vi "檔案管理.vi"() -> ()   [LabVIEW 2015]
uses:
  Control_cluster_IOConstant.ctl
  C:/Users/jeff.lin.MINAIK/Desktop/Scripting/Control_MessageCluster.ctl
  <userlib>/FGV/control/Control_Data.ctl
panel:
  out "Array 2":string[](array[string])
  in  "Listbox":i32(listbox)
  out "error out":errorcluster
  in  "ProjectName":string
  in  "Project":string(combo)
  in  "file (use dialog)":path=path "D:/dataFGV"
  in  "重新載入":bool
  out "Array":cluster{"Name":string, "Cluster In 2":T1}[](array[cluster])
  in  "Cluster In":T1
  out "Cluster Out":cluster{"Name":string, "Cluster In 2":T1}
  in  "儲存檔案":bool
  in  "匯入檔案":bool
  in  "開啟檔案":bool
  in  "檔案初始化":bool
  in  "更新資料":bool
  in  "刪除資料":bool
  in  "插入資料":bool
  in  "增加資料":bool
  in  "儲存資料":bool
  in  "讀取資料":bool
  in  "資料初始化":bool
  in  "離開":bool
  in  "等待":bool
  in  "系統初始化":bool
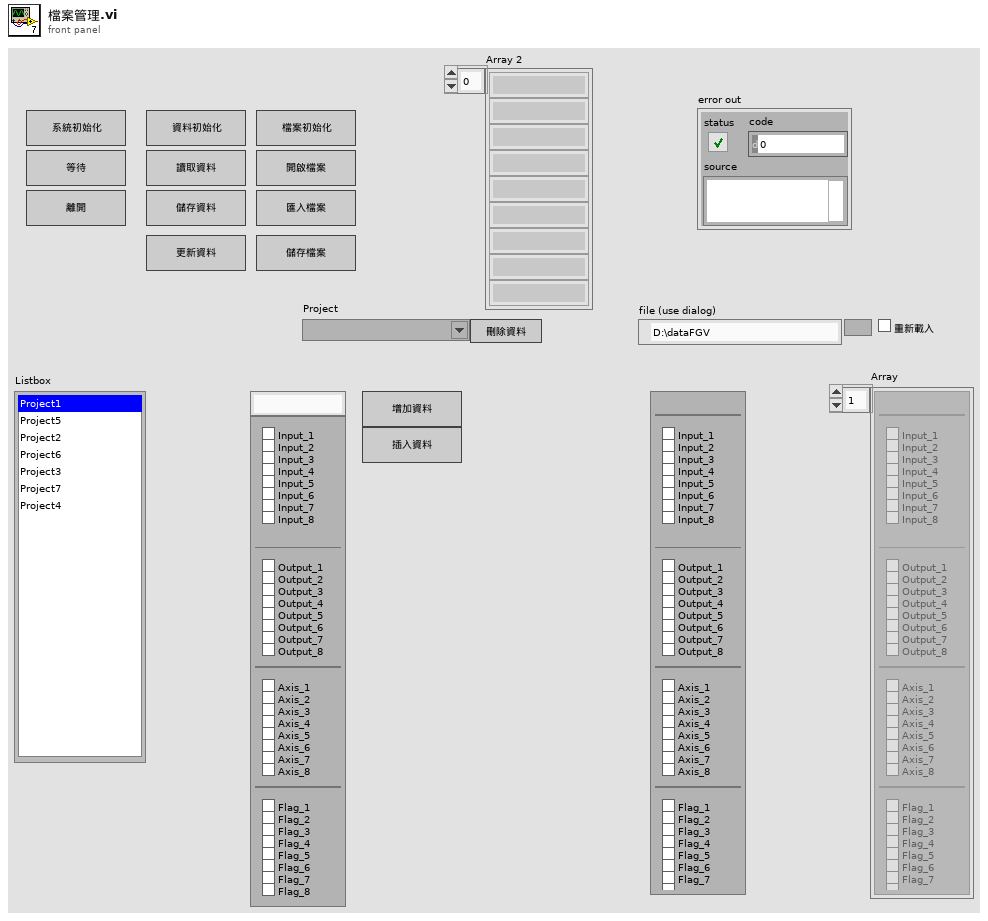
[diagram p1: front panel]
types:
  T1 = typedef "Control_cluster_IOConstant.ctl" = cluster{"Cluster_Input":cluster{"Input1":bool, "Input2":bool, "Input3":bool, "Input4":bool, "Input5":bool, "Input6":bool, "Input7":bool, "Input8":bool}, "Cluster_Output":cluster{"Output8":bool, "Output7":bool, "Output6":bool, "Output5":bool, "Output4":bool, "Output3":bool, "Output2":bool, "Output1":bool}, "Cluster_Axis":cluster{"Axis1":bool, "Axis2":bool, "Axis3":bool, "Axis4":bool, "Axis5":bool, "Axis6":bool, "Axis7":bool, "Axis8":bool}, "Cluster_Flag":cluster{"Flag1":bool, "Flag2":bool, "Flag3":bool, "Flag4":bool, "Flag5":bool, "Flag6":bool, "Flag7":bool, "Flag8":bool}}
  T2 = typedef "Control_Data.ctl" = enum16{"Initialize", "Get Data", "Set Data", "Delete Data", "Idle"}
  T3 = typedef "Control_MessageCluster.ctl" = cluster{"Message":string, "Message Data":variant}
  T4 = typedef "Control_enum_檔案控制.ctl" = enum16{"檔案初始化", "開啟檔案", "匯入檔案", "儲存檔案"}
  T5 = typedef "Control_enum_資料控制.ctl" = enum16{"資料初始化", "讀取資料", "儲存資料", "增加資料", "插入資料", "刪除資料", "更新資料"}
  T6 = typedef "Control_enum_系統.ctl" = enum16{"系統初始化", "等待", "離開"}
  T7 = cluster{"Data name":string, "Data In":cluster{"Data name":string, "Data":variant}}
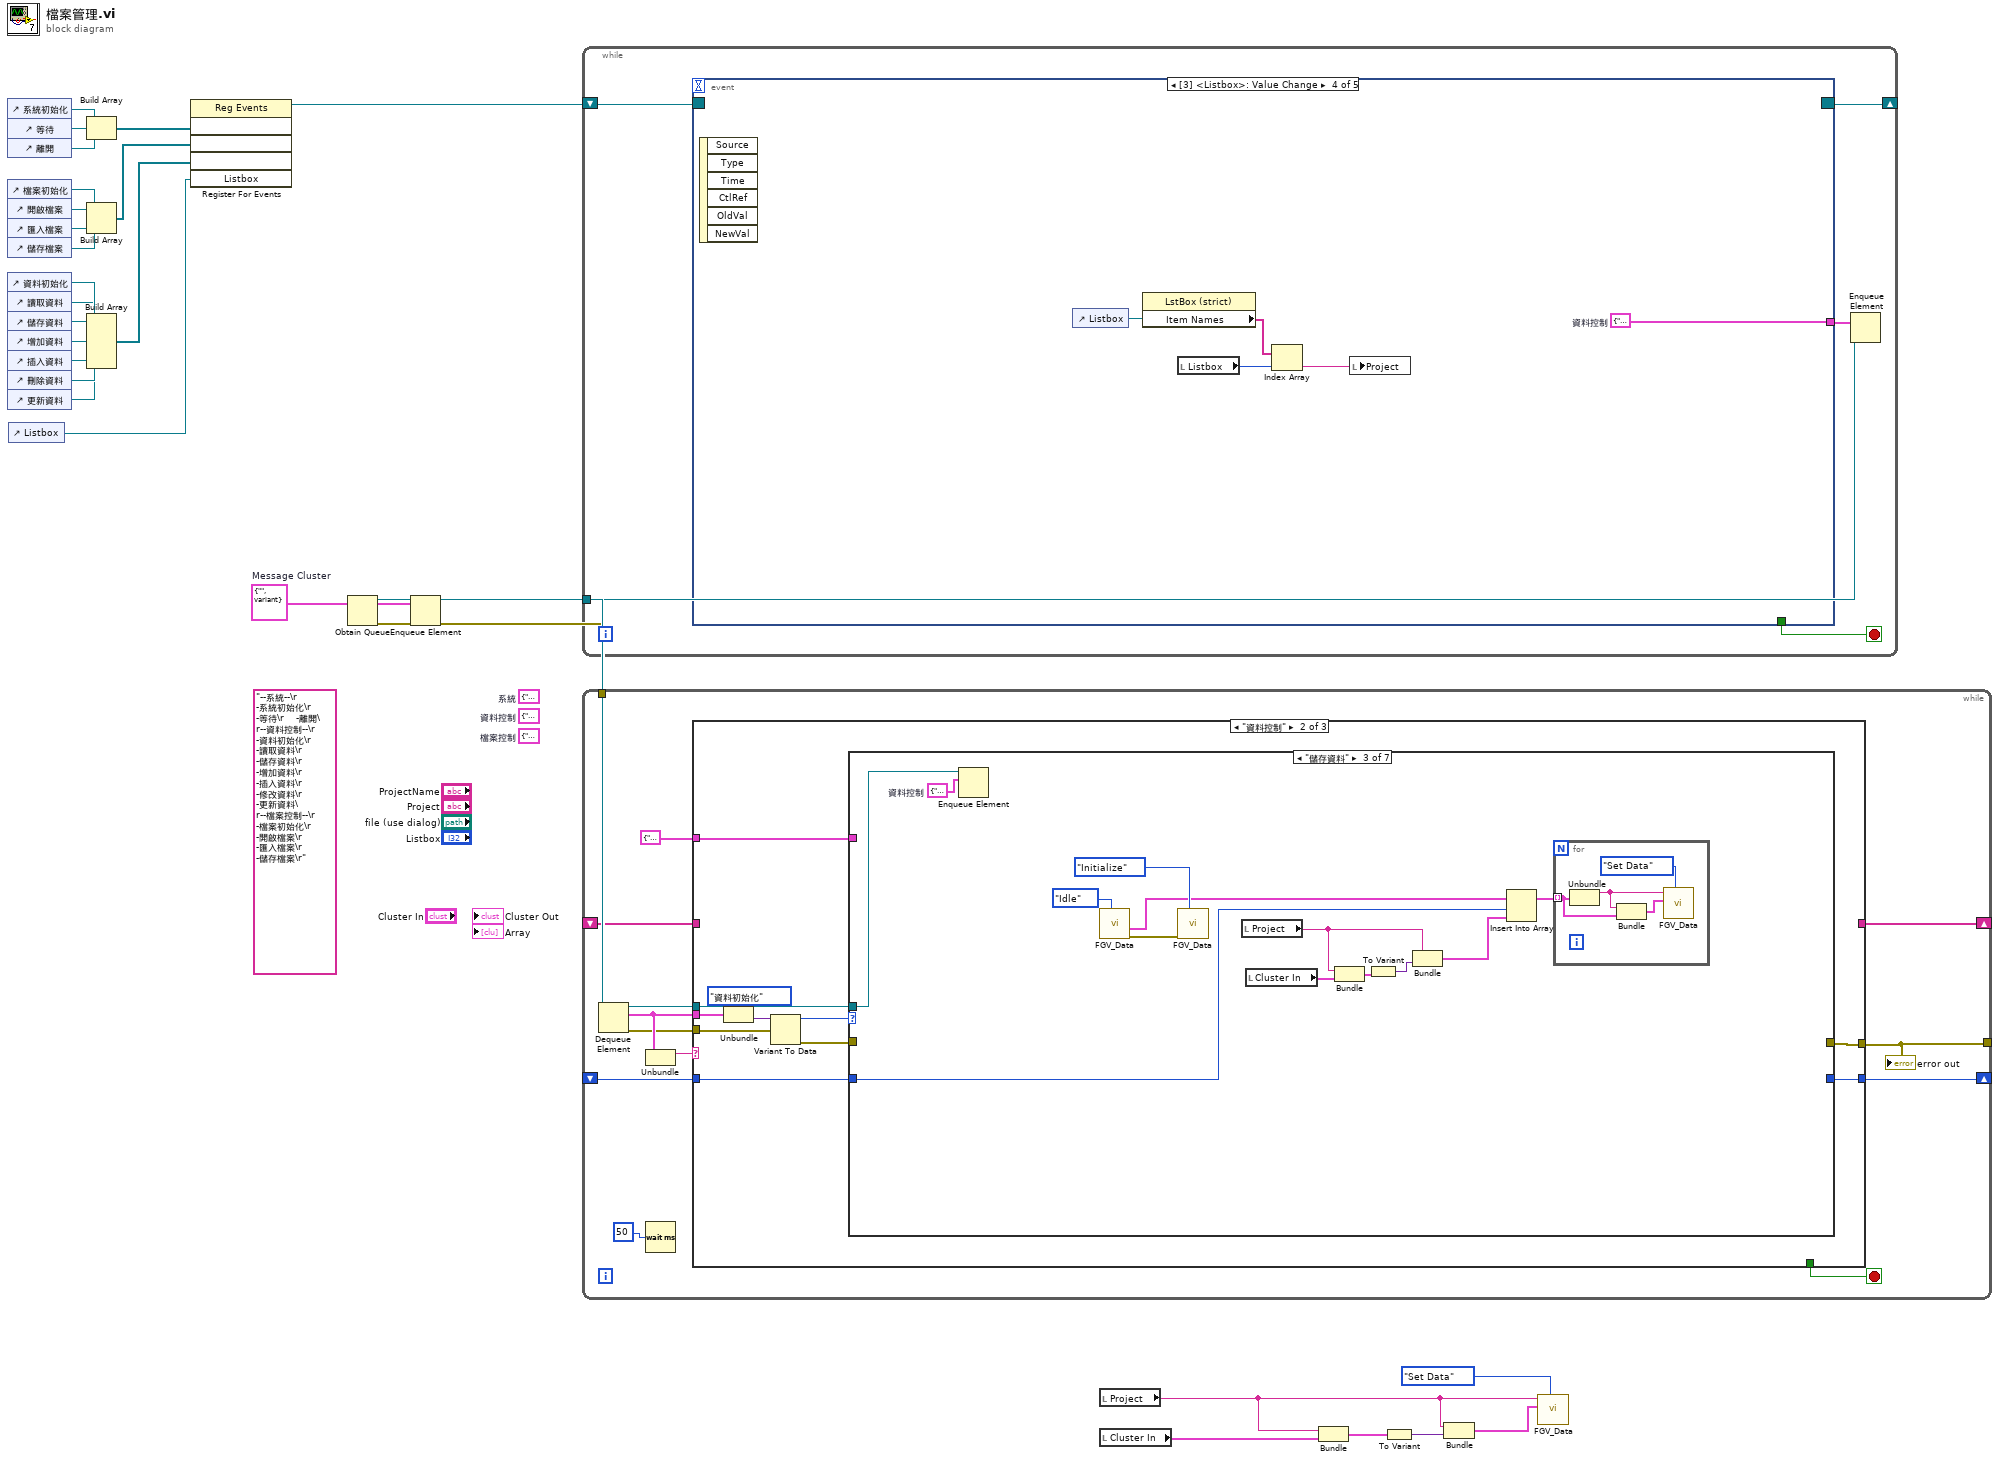
[diagram p0: block diagram]
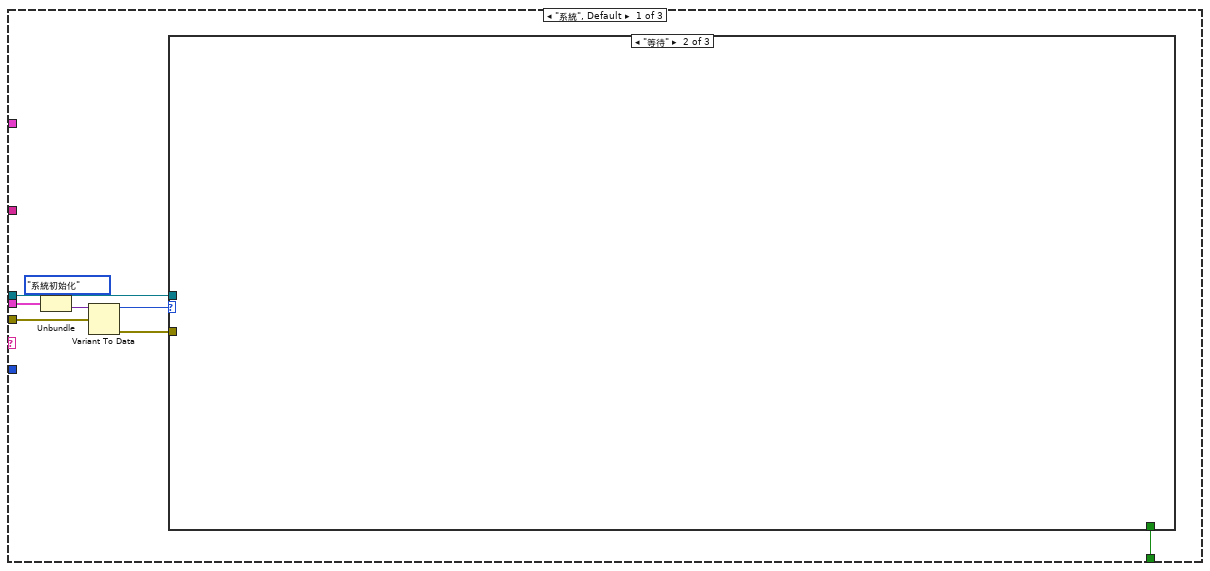
[diagram p2: hidden frame]
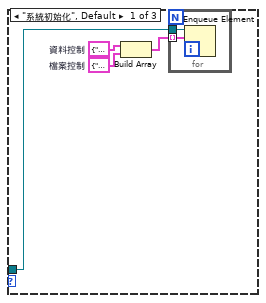
[diagram p3: hidden frame]
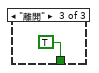
[diagram p4: hidden frame]
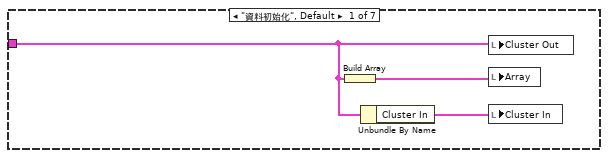
[diagram p5: hidden frame]
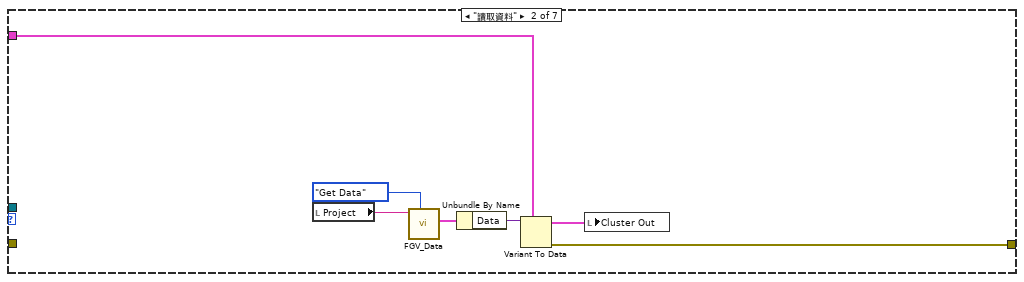
[diagram p6: hidden frame]
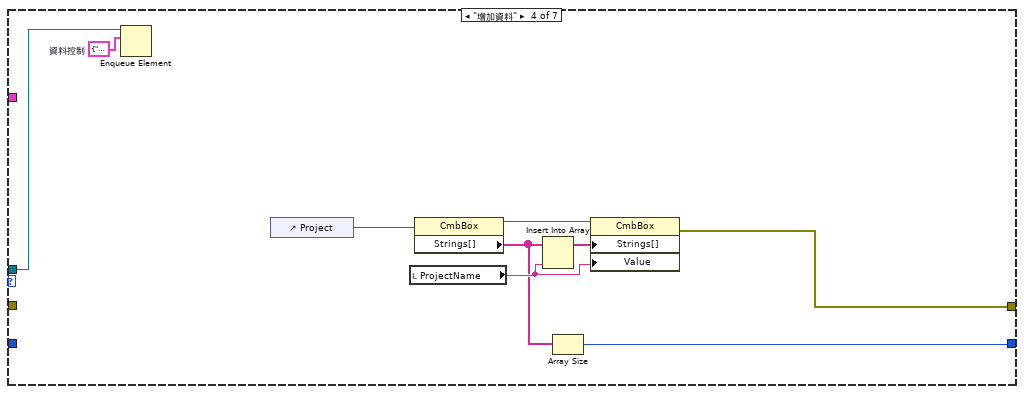
[diagram p7: hidden frame]
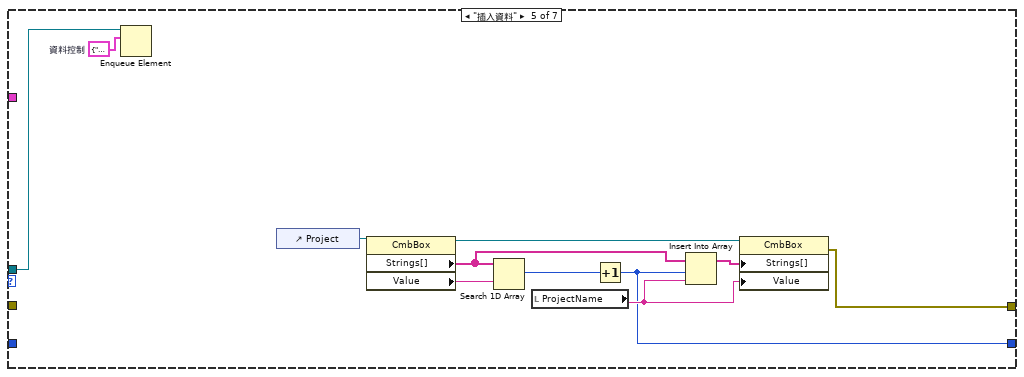
[diagram p8: hidden frame]
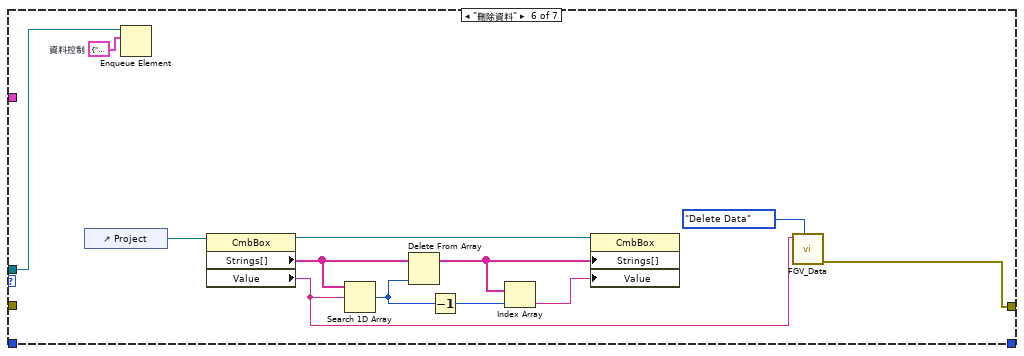
[diagram p9: hidden frame]
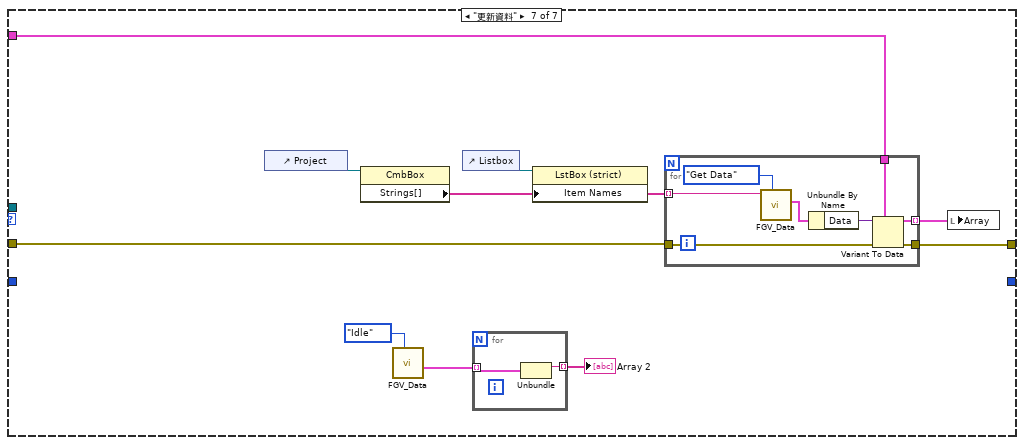
[diagram p10: hidden frame]
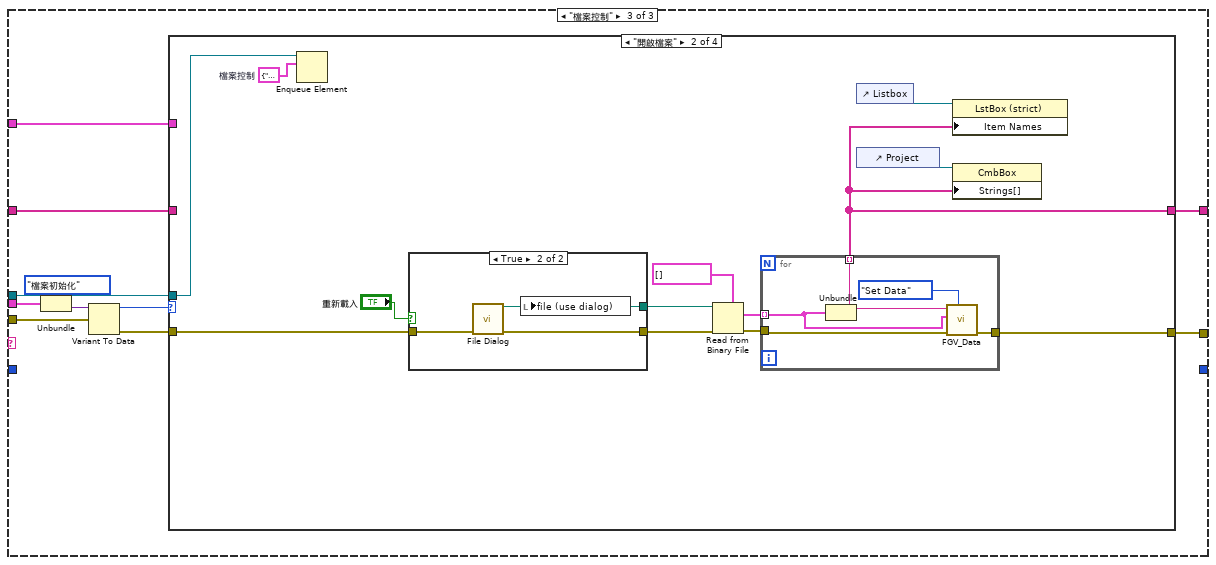
[diagram p11: hidden frame]
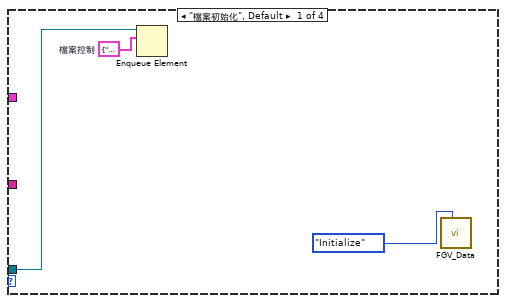
[diagram p12: hidden frame]
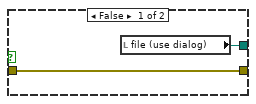
[diagram p13: hidden frame]
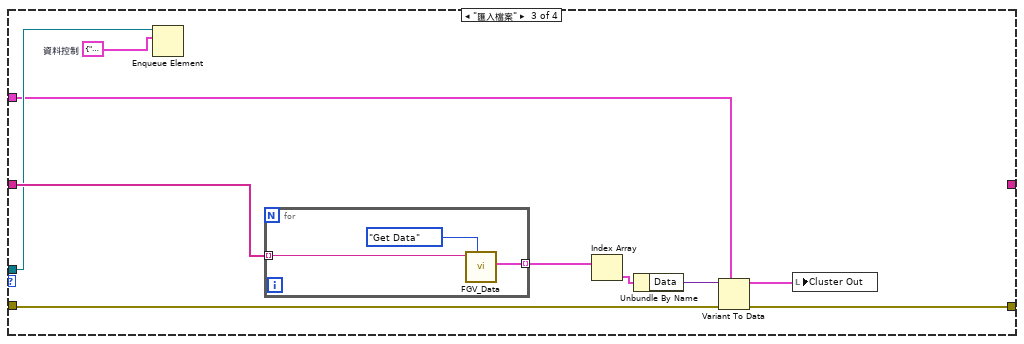
[diagram p14: hidden frame]
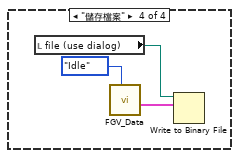
[diagram p15: hidden frame]
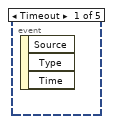
[diagram p16: hidden frame]
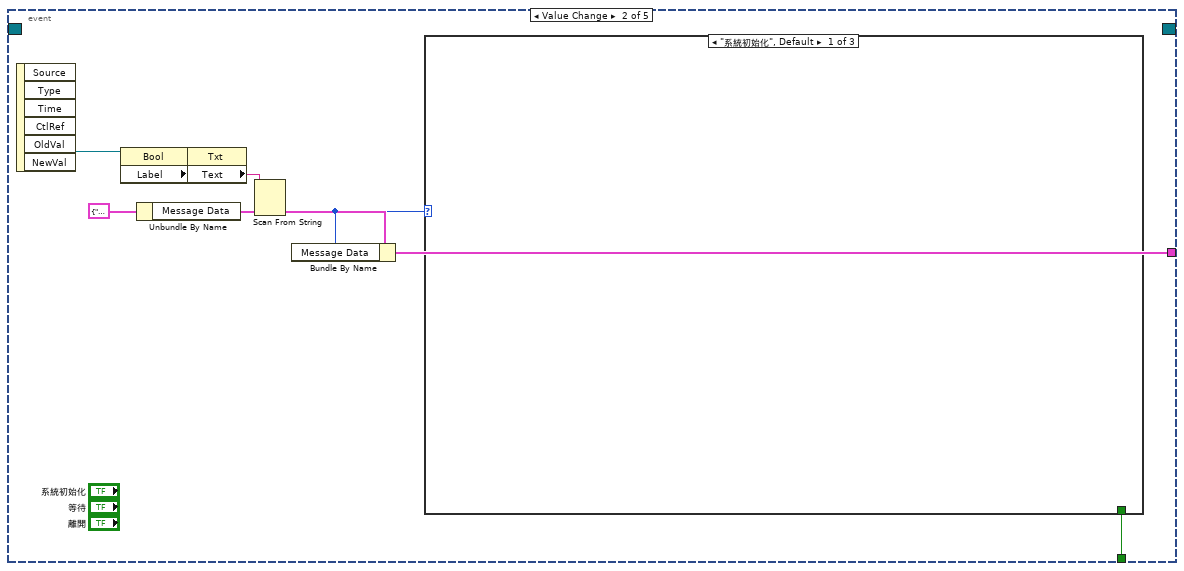
[diagram p17: hidden frame]
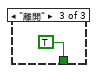
[diagram p19: hidden frame]
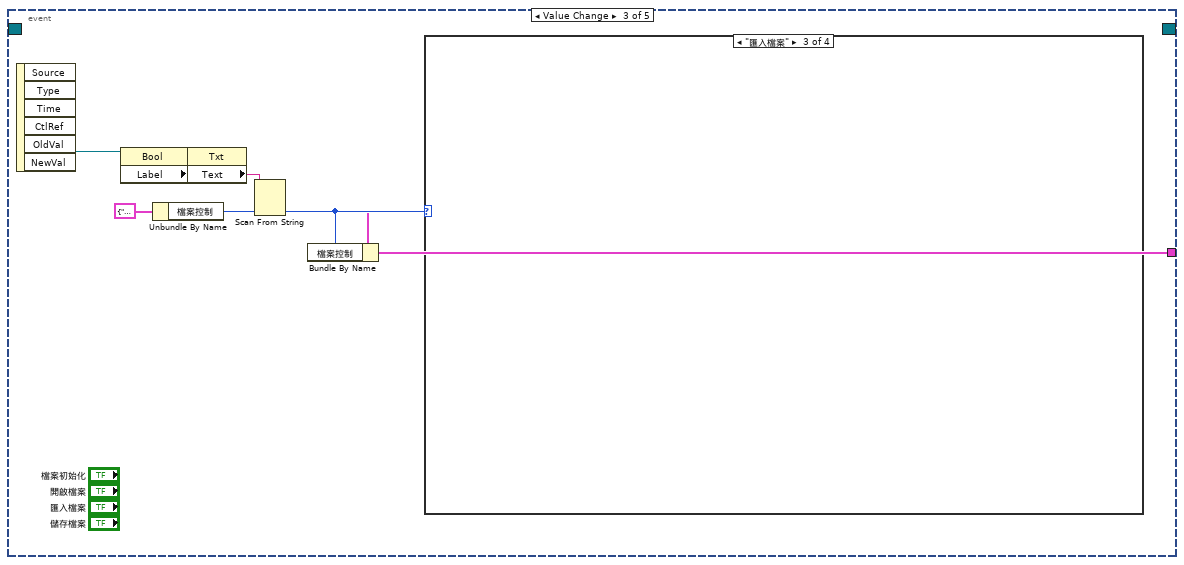
[diagram p20: hidden frame]
diagram:
  w30 = T3 {"Message"="", "Message Data"=variant}  # Message Cluster
  (unwired) "--系統--\r    -系統初始化\r    -等待\r    -離開\r--資料控制--\r    -資料初始化\r    -讀取資料\r    -儲存資料\r    -增加資料\r    -插入資料\r    -修改資料\r    -更新資料\r--檔案控制--\r    -檔案初始化\r    -開啟檔案\r    -匯入檔案\r    -儲存檔案\r"
  (unwired) cluster{"Message":string, "檔案控制":T4} {"Message"="檔案控制", "檔案控制"=enum."檔案初始化"}  # 檔案控制
  (unwired) cluster{"Message":string, "資料控制":T5} {"Message"="資料控制", "資料控制"=enum."資料初始化"}  # 資料控制
  (unwired) cluster{"Message":string, "系統":T6} {"Message"="系統", "系統"=enum."系統初始化"}  # 系統
  n1 = control-ref of="系統初始化"() -> (w27:refnum<vi>)
  n2 = control-ref of="等待"() -> (w26:refnum<vi>)
  n3 = control-ref of="離開"() -> (w25:refnum<vi>)
  n4 = control-ref of="檔案初始化"() -> (w13:refnum<vi>)
  n5 = control-ref of="開啟檔案"() -> (w12:refnum<vi>)
  n6 = control-ref of="匯入檔案"() -> (w11:refnum<vi>)
  n7 = control-ref of="儲存檔案"() -> (w10:refnum<vi>)
  n8 = control-ref of="資料初始化"() -> (w20:refnum<vi>)
  n9 = control-ref of="讀取資料"() -> (w19:refnum<vi>)
  n10 = control-ref of="儲存資料"() -> (w18:refnum<vi>)
  n11 = control-ref of="增加資料"() -> (w17:refnum<vi>)
  n12 = control-ref of="插入資料"() -> (w16:refnum<vi>)
  n13 = control-ref of="刪除資料"() -> (w15:refnum<vi>)
  n14 = control-ref of="更新資料"() -> (w14:refnum<vi>)
  n15 = control-ref of="Listbox"() -> (w7:refnum<vi>)
  n16 = Build Array(w27, w26, w25) -> (w24:refnum<vi>[])
  n17 = Build Array(w13, w12, w11, w10) -> (w9:refnum<vi>[])
  n18 = Build Array(w20, w19, w18, w17, w16, w15, w14) -> (w8:refnum<vi>[])
  n19 = register-events(w24, w9, w8, w7) -> (reference out=w23:refnum<event-registration>)  [unwired: 2 in, 1 out]
  n20 = Obtain Queue(element data type=w30) -> (queue out=w28:refnum<queue>, error out=w29:errorcluster)  [unwired: 4 in, 1 out]
  n21 = Enqueue Element(queue=w28, element=w30, error in (no error)=w29) -> (queue out=w22:refnum<queue>, error out=w21:errorcluster)  [unwired: 1 in, 1 out]
  n22 = while {
    shift-right: [w35] -> _
    shift-left: w23 -> [w34]
    tunnel: w22 -> [w32]
    stop <- w31 stop-if-true
    n23 = event shown="[3] <Listbox>: Value Change" {
      selector: w34 -> [_ _ _ _ _]
      dyn-events: [_ _ _ _ _] -> w35
      timeout: _ -> [_ _ _ _ _]
      tunnel: [_ w37 w45 w56 w57] -> w33
      tunnel: [_ w36 _ _ _] -> w31
      event Timeout {
        n24 = event-data() -> ()  [unwired: 1 in, 3 out]
      }
      event Value Change {
        w41 = cluster{"Message":string, "Message Data":T6} {"Message"="系統", "Message Data"=enum."系統初始化"} ("系統")
        n25 = event-data() -> ("CtlRef"=w43:refnum<vi>)  [unwired: 1 in, 5 out]
        n26 = property class="Bool"(reference=w43) -> ("Label"=w42:refnum<vi>)  [unwired: 1 in, 2 out]
        n27 = Unbundle By Name(w41) -> ("Message Data"=w40:T6)
        n28 = property class="Txt"(reference=w42) -> ("Text"=w39:string)  [unwired: 1 in, 2 out]
        n29 = Scan From String(input string=w39, default 1=w40) -> (output 1=w38:T6)  [unwired: 3 in, 3 out]
        n30 = Bundle By Name(cluster=w41, "Message Data"=w38) -> (w37:cluster{"Message":string, "Message Data":T6})
        n31 = case shown="\"系統初始化\", Default" w38 {
          tunnel: [_ _ TRUE] -> w36
          frame "系統初始化", Default {
          }
          frame "等待" {
          }
          frame "離開" {
          }
        }
      }
      event Value Change {
        w46 = cluster{"Message":string, "檔案控制":T4} {"Message"="檔案控制", "檔案控制"=enum."檔案初始化"} ("檔案控制")
        n32 = event-data() -> ("CtlRef"=w47:refnum<vi>)  [unwired: 1 in, 5 out]
        n33 = property class="Bool"(reference=w47) -> ("Label"=w51:refnum<vi>)  [unwired: 1 in, 2 out]
        n34 = Unbundle By Name(w46) -> ("檔案控制"=w50:T4)
        n35 = property class="Txt"(reference=w51) -> ("Text"=w49:string)  [unwired: 1 in, 2 out]
        n36 = Scan From String(input string=w49, default 1=w50) -> (output 1=w48:T4)  [unwired: 3 in, 3 out]
        n37 = Bundle By Name(cluster=w46, "檔案控制"=w48) -> (w45:cluster{"Message":string, "檔案控制":T4})
        n38 = case shown="\"匯入檔案\"" w48 {
          frame "檔案初始化", Default {
          }
          frame "開啟檔案" {
          }
          frame "匯入檔案" {
          }
          frame "儲存檔案" {
          }
        }
      }
      event Value Change {
        w56 = cluster{"Message":string, "資料控制":T5} {"Message"="資料控制", "資料控制"=enum."讀取資料"}  # 資料控制
        n39 = event-data() -> ()  [unwired: 1 in, 6 out]
        n40 = control-ref of="Listbox"() -> (w55:refnum<vi>)
        n41 = property class="LstBox (strict)"(reference=w55) -> ("Item Names"=w53:string[])  [unwired: 1 in, 2 out]
        n42 = local read "Listbox"() -> (w54:i32)
        n43 = Index Array(array=w53, index=w54) -> (element=w52:string)
        n44 = local write "Project"(w52) -> ()
      }
      event Value Change {
        w58 = cluster{"Message":string, "資料控制":T5} {"Message"="資料控制", "資料控制"=enum."資料初始化"}  # 資料控制
        n45 = event-data() -> ("CtlRef"=w59:refnum<vi>)  [unwired: 1 in, 5 out]
        n46 = property class="Bool"(reference=w59) -> ("Label"=w63:refnum<vi>)  [unwired: 1 in, 2 out]
        n47 = Unbundle By Name(w58) -> ("資料控制"=w62:T5)
        n48 = property class="Txt"(reference=w63) -> ("Text"=w61:string)  [unwired: 1 in, 2 out]
        n49 = Scan From String(input string=w61, default 1=w62) -> (output 1=w60:T5)  [unwired: 3 in, 3 out]
        n50 = Bundle By Name(cluster=w58, "資料控制"=w60) -> (w57:cluster{"Message":string, "資料控制":T5})
        n51 = case shown="\"插入資料\"" w60 {
          frame "資料初始化", Default {
          }
          frame "讀取資料" {
          }
          frame "儲存資料" {
          }
          frame "增加資料" {
          }
          frame "插入資料" {
          }
          frame "刪除資料" {
          }
          frame "更新資料" {
          }
        }
      }
    }
    n52 = Enqueue Element(queue=w32, element=w33) -> ()  [unwired: 2 in, 3 out]
  }
  n53 = while {
    tunnel: w22 -> [w77]
    tunnel: w21 -> [w76]
    shift-right: [w69] -> _
    shift-left: _ -> [w70]
    tunnel: [w68] -> _
    shift-right: [w65] -> _
    shift-left: _ -> [w64]
    stop <- w71 stop-if-true
    n54 = Dequeue Element(queue=w77, error in (no error)=w76) -> (queue out=w72:refnum<queue>, element=w74:T3, error out=w73:errorcluster)  [unwired: 1 in, 1 out]
    n55 = Unbundle(w74) -> ("Message"=w75:string)  [unwired: 1 out]
    n56 = Wait (ms)(milliseconds to wait=50) -> ()  [unwired: 1 out]
    n57 = case shown="\"資料控制\"" w75 {
      tunnel: w74 -> [w85 w103 w193]
      tunnel: w73 -> [w83 w101 w191]
      tunnel: w72 -> [w79 w97 w187]
      tunnel: [w78 _ _] -> w71
      tunnel: w70 -> [_ _ w186]
      tunnel: [_ _ w185] -> w69
      tunnel: [_ w96 w184] -> w68
      tunnel: cluster{"Name":string, "Cluster In":T1} {"Name"="", "Cluster In"={"Cluster_Input"={"Input1"=FALSE, "Input2"=FALSE, "Input3"=FALSE, "Input4"=FALSE, "Input5"=FALSE, "Input6"=FALSE, "Input7"=FALSE, "Input8"=FALSE}, "Cluster_Output"={"Output8"=FALSE, "Output7"=FALSE, "Output6"=FALSE, "Output5"=FALSE, "Output4"=FALSE, "Output3"=FALSE, "Output2"=FALSE, "Output1"=FALSE}, "Cluster_Axis"={"Axis1"=FALSE, "Axis2"=FALSE, "Axis3"=FALSE, "Axis4"=FALSE, "Axis5"=FALSE, "Axis6"=FALSE, "Axis7"=FALSE, "Axis8"=FALSE}, "Cluster_Flag"={"Flag1"=FALSE, "Flag2"=FALSE, "Flag3"=FALSE, "Flag4"=FALSE, "Flag5"=FALSE, "Flag6"=FALSE, "Flag7"=FALSE, "Flag8"=FALSE}}} ("Cluster Out 2") -> [_ w95 w183]
      tunnel: [_ w94 _] -> w65
      tunnel: w64 -> [_ w93 _]
      frame "系統", Default {
        n58 = Unbundle(w85) -> ("Message Data"=w84:variant)  [unwired: 1 out]
        n59 = Variant To Data(error in=w83, type=Control_enum_系統."系統初始化" ("系統"), Variant=w84) -> (data=w81:T6, error out=w80:errorcluster)
        n60 = case shown="\"等待\"" w81 {
          tunnel: w80 -> [_ _ _]
          tunnel: w79 -> [w86 _ _]
          tunnel: [_ _ TRUE] -> w78
          frame "系統初始化", Default {
            w89 = cluster{"Message":string, "檔案控制":T4} {"Message"="檔案控制", "檔案控制"=enum."檔案初始化"}  # 檔案控制
            w88 = cluster{"Message":string, "資料控制":T5} {"Message"="資料控制", "資料控制"=enum."資料初始化"}  # 資料控制
            n61 = Build Array(w88, w89) -> (w87:cluster{"Message":string, "檔案控制":u16}[])
            n62 = for {
              tunnel: w87 -> [w91] mode=indexing
              tunnel: w86 -> [w90]
              n63 = Enqueue Element(queue=w90, element=w91) -> ()  [unwired: 2 in, 3 out]
            }
          }
          frame "等待" {
          }
          frame "離開" {
          }
        }
      }
      frame "資料控制" {
        n64 = Unbundle(w103) -> ("Message Data"=w102:variant)  [unwired: 1 out]
        n65 = Variant To Data(error in=w101, type=Control_enum_資料控制."資料初始化" ("資料控制"), Variant=w102) -> (data=w99:T5, error out=w98:errorcluster)
        n66 = case shown="\"儲存資料\"" w99 {
          tunnel: w98 -> [_ _ _ _ _ _ w172]
          tunnel: w97 -> [_ _ w124 w134 w145 w155 _]
          tunnel: w95 -> [w105 w108 _ _ _ _ w171]
          tunnel: [_ w107 _ w133 w142 w153 w170] -> w96
          tunnel: [_ _ _ w131 w140 _ _] -> w94
          tunnel: w93 -> [_ _ w115 _ _ _ _]
          frame "資料初始化", Default {
            n67 = Build Array(w105) -> (w106:cluster{"Name":string, "Cluster In":T1}[])
            n68 = Unbundle By Name(w105) -> ("Cluster In"=w104:T1)
            n69 = local write "Cluster Out"(w105) -> ()
            n70 = local write "Array"(w106) -> ()
            n71 = local write "Cluster In"(w104) -> ()
          }
          frame "讀取資料" {
            n72 = local read "Project"() -> (w109:string)
            n73 = call <userlib>:"FGV_Data.vi"("Action_Data"=Control_Data."Get Data", "Data name"=w109) -> ("Data  Out"=w110:cluster{"Data name":string, "Data":variant})  [unwired: 6 in, 3 out]
            n74 = Unbundle By Name(w110) -> ("Data"=w112:variant)
            n75 = Variant To Data(type=w108, Variant=w112) -> (data=w111:cluster{"Name":string, "Cluster In":T1}, error out=w107:errorcluster)  [unwired: 1 in]
            n76 = local write "Cluster Out"(w111) -> ()
          }
          frame "儲存資料" {
            w125 = cluster{"Message":string, "資料控制":T5} {"Message"="資料控制", "資料控制"=enum."更新資料"}  # 資料控制
            n77 = Enqueue Element(queue=w124, element=w125) -> ()  [unwired: 2 in, 3 out]
            n78 = call <userlib>:"FGV_Data.vi"("Action_Data"=Control_Data."Idle") -> ("error out"=w119:errorcluster, "Data Array out"=w117:cluster{"Data name":string, "Data":variant}[])  [unwired: 7 in, 2 out]
            n79 = call <userlib>:"FGV_Data.vi"("Action_Data"=Control_Data."Initialize", "error in"=w119) -> ()  [unwired: 6 in, 4 out]
            n80 = local read "Project"() -> (w121:string)
            n81 = local read "Cluster In"() -> (w122:T1)
            n82 = Bundle("Project"=w121, "Cluster In"=w122) -> (w123:cluster{"Project":string, "Cluster In":T1})  [unwired: 1 in]
            n83 = To Variant(anything=w123) -> (Variant=w126:variant)
            n84 = Bundle("Project"=w121, "Variant"=w126) -> (w114:cluster{"Project":string, "Variant":variant})  [unwired: 1 in]
            n85 = Insert Into Array(array=w117, index=w115, new element=w114) -> (w116:cluster{"Data name":string, "Data":variant}[])
            n86 = for {
              tunnel: w116 -> [w129] mode=indexing
              n87 = Unbundle(w129) -> ("Data name"=w127:string)  [unwired: 1 out]
              n88 = Bundle("Data name"=w127, "Data In"=w129) -> (w128:T7)  [unwired: 1 in]
              n89 = call <userlib>:"FGV_Data.vi"("Action_Data"=Control_Data."Set Data", "Data In"=w128, "Data name"=w127) -> ()  [unwired: 5 in, 4 out]
            }
          }
          frame "增加資料" {
            w135 = cluster{"Message":string, "資料控制":T5} {"Message"="資料控制", "資料控制"=enum."儲存資料"}  # 資料控制
            n90 = Enqueue Element(queue=w134, element=w135) -> ()  [unwired: 2 in, 3 out]
            n91 = control-ref of="Project"() -> (w138:refnum<vi>)
            n92 = local read "ProjectName"() -> (w136:string)
            n93 = property class="CmbBox"(reference=w138) -> (reference out=w137:refnum<vi>, "Strings[]"=w132:string[])  [unwired: 1 in, 1 out]
            n94 = Insert Into Array(array=w132, new element=w136) -> (w139:string[])  [unwired: 1 in]
            n95 = Array Size(array=w132) -> (size(s)=w131:i32)
            n96 = property class="CmbBox"(reference=w137, "Strings[]"=w139, "Value"=w136) -> (error out=w133:errorcluster)  [unwired: 1 in, 1 out]
          }
          frame "插入資料" {
            w146 = cluster{"Message":string, "資料控制":T5} {"Message"="資料控制", "資料控制"=enum."儲存資料"}  # 資料控制
            n97 = Enqueue Element(queue=w145, element=w146) -> ()  [unwired: 2 in, 3 out]
            n98 = control-ref of="Project"() -> (w148:refnum<vi>)
            n99 = property class="CmbBox"(reference=w148) -> (reference out=w149:refnum<vi>, "Strings[]"=w144:string[], "Value"=w147:string)  [unwired: 1 in, 1 out]
            n100 = Search 1D Array(1D array=w144, element=w147) -> (index of element=w143:i32)  [unwired: 1 in]
            n101 = local read "ProjectName"() -> (w141:string)
            n102 = Increment(x=w143) -> (x+1=w140:i32)
            n103 = Insert Into Array(array=w144, index=w140, new element=w141) -> (w150:string[])
            n104 = property class="CmbBox"(reference=w149, "Strings[]"=w150, "Value"=w141) -> (error out=w142:errorcluster)  [unwired: 1 in, 1 out]
          }
          frame "刪除資料" {
            w154 = cluster{"Message":string, "資料控制":T5} {"Message"="資料控制", "資料控制"=enum."更新資料"}  # 資料控制
            n105 = control-ref of="Project"() -> (w156:refnum<vi>)
            n106 = Enqueue Element(queue=w155, element=w154) -> ()  [unwired: 2 in, 3 out]
            n107 = property class="CmbBox"(reference=w156) -> (reference out=w162:refnum<vi>, "Strings[]"=w161:string[], "Value"=w159:string)  [unwired: 1 in, 1 out]
            n108 = Search 1D Array(1D array=w161, element=w159) -> (index of element=w152:i32)  [unwired: 1 in]
            n109 = Delete From Array(array=w161, index=w152) -> (array with subset deleted=w158:string[])  [unwired: 1 in, 1 out]
            n110 = Decrement(x=w152) -> (x-1=w151:i32)
            n111 = Index Array(array=w158, index=w151) -> (element=w157:string)
            n112 = property class="CmbBox"(reference=w162, "Strings[]"=w158, "Value"=w157) -> ()  [unwired: 1 in, 2 out]
            n113 = call <userlib>:"FGV_Data.vi"("Action_Data"=Control_Data."Delete Data", "Data name"=w159) -> ("error out"=w153:errorcluster)  [unwired: 6 in, 3 out]
          }
          frame "更新資料" {
            n114 = control-ref of="Project"() -> (w167:refnum<vi>)
            n115 = property class="CmbBox"(reference=w167) -> ("Strings[]"=w166:string[])  [unwired: 1 in, 2 out]
            n116 = call <userlib>:"FGV_Data.vi"("Action_Data"=Control_Data."Idle") -> ("Data Array out"=w164:cluster{"Data name":string, "Data":variant}[])  [unwired: 7 in, 3 out]
            n117 = control-ref of="Listbox"() -> (w169:refnum<vi>)
            n118 = for {
              tunnel: w164 -> [w174] mode=indexing
              tunnel: [w173] -> w163 mode=indexing
              n119 = Unbundle(w174) -> ("Data name"=w173:string)  [unwired: 1 out]
            }
            "Array 2" <- w163
            n120 = property class="LstBox (strict)"(reference=w169, "Item Names"=w166) -> ()  [unwired: 1 in, 2 out]
            n121 = for {
              tunnel: w172 -> [w180]
              tunnel: w166 -> [w179] mode=indexing
              tunnel: [w177] -> w168 mode=indexing
              tunnel: w171 -> [w176]
              tunnel: [w175] -> w170
              n122 = call <userlib>:"FGV_Data.vi"("Action_Data"=Control_Data."Get Data", "Data name"=w179) -> ("Data  Out"=w178:cluster{"Data name":string, "Data":variant})  [unwired: 6 in, 3 out]
              n123 = Unbundle By Name(w178) -> ("Data"=w181:variant)
              n124 = Variant To Data(error in=w180, type=w176, Variant=w181) -> (data=w177:cluster{"Name":string, "Cluster In":T1}, error out=w175:errorcluster)
            }
            n125 = local write "Array"(w168) -> ()
          }
        }
      }
      frame "檔案控制" {
        n126 = Unbundle(w193) -> ("Message Data"=w192:variant)  [unwired: 1 out]
        n127 = Variant To Data(error in=w191, type=Control_enum_檔案控制."檔案初始化" ("檔案控制"), Variant=w192) -> (data=w189:T4, error out=w188:errorcluster)
        n128 = case shown="\"開啟檔案\"" w189 {
          tunnel: w188 -> [_ w204 w225 _]
          tunnel: w187 -> [w196 w203 w222 _]
          tunnel: w186 -> [_ _ w224 _]
          tunnel: [_ w197 _ _] -> w185
          tunnel: [_ w201 w223 _] -> w184
          tunnel: w183 -> [_ _ w220 _]
          frame "檔案初始化", Default {
            w194 = cluster{"Message":string, "檔案控制":T4} {"Message"="檔案控制", "檔案控制"=enum."開啟檔案"}  # 檔案控制
            n129 = Enqueue Element(queue=w196, element=w194) -> ()  [unwired: 2 in, 3 out]
            n130 = call <userlib>:"FGV_Data.vi"("Action_Data"=Control_Data."Initialize") -> ()  [unwired: 7 in, 4 out]
          }
          frame "開啟檔案" {
            w202 = cluster{"Message":string, "檔案控制":T4} {"Message"="檔案控制", "檔案控制"=enum."匯入檔案"}  # 檔案控制
            n131 = Enqueue Element(queue=w203, element=w202) -> ()  [unwired: 2 in, 3 out]
            n132 = case shown="True" "重新載入" {
              tunnel: [w210 w212] -> w207
              tunnel: w204 -> [w211 w214]
              tunnel: [w211 w213] -> w208
              frame False {
                n133 = local read "file (use dialog)"() -> (w210:path)
              }
              frame True {
                n134 = call "File Dialog"("error in"=w214) -> ("selected path"=w212:path, "error out"=w213:errorcluster)  [unwired: 11 in, 2 out]
                n135 = local write "file (use dialog)"(w212) -> ()
              }
            }
            n136 = Read from Binary File(5:cluster{"Data name":string, "Data":variant}[] [] ("Data Array out"), 8:w208, 11:w207) -> (0:w205:errorcluster, 2:w206:cluster{"Data name":string, "Data":variant}[])  [unwired: 3 in, 2 out]
            n137 = for {
              tunnel: w206 -> [w219] mode=indexing
              tunnel: w205 -> [w215]
              tunnel: [w217] -> w197 mode=indexing
              tunnel: [w216] -> w201
              n138 = Unbundle(w219) -> ("Data name"=w217:string)  [unwired: 1 out]
              n139 = call <userlib>:"FGV_Data.vi"("Action_Data"=Control_Data."Set Data", "error in"=w215, "Data In"=w219, "Data name"=w217) -> ("error out"=w216:errorcluster)  [unwired: 4 in, 3 out]
            }
            n140 = control-ref of="Listbox"() -> (w198:refnum<vi>)
            n141 = control-ref of="Project"() -> (w199:refnum<vi>)
            n142 = property class="LstBox (strict)"(reference=w198, "Item Names"=w197) -> ()  [unwired: 1 in, 2 out]
            n143 = property class="CmbBox"(reference=w199, "Strings[]"=w197) -> ()  [unwired: 1 in, 2 out]
          }
          frame "匯入檔案" {
            w221 = cluster{"Message":string, "資料控制":T5} {"Message"="資料控制", "資料控制"=enum."更新資料"}  # 資料控制
            n144 = Enqueue Element(queue=w222, element=w221) -> ()  [unwired: 2 in, 3 out]
            n145 = for {
              tunnel: w224 -> [w231] mode=indexing
              tunnel: [w230] -> w229 mode=indexing
              n146 = call <userlib>:"FGV_Data.vi"("Action_Data"=Control_Data."Get Data", "Data name"=w231) -> ("Data  Out"=w230:cluster{"Data name":string, "Data":variant})  [unwired: 6 in, 3 out]
            }
            n147 = Index Array(array=w229) -> (element=w226:cluster{"Data name":string, "Data":variant})  [unwired: 1 in]
            n148 = Unbundle By Name(w226) -> ("Data"=w227:variant)
            n149 = Variant To Data(error in=w225, type=w220, Variant=w227) -> (data=w228:cluster{"Name":string, "Cluster In":T1}, error out=w223:errorcluster)
            n150 = local write "Cluster Out"(w228) -> ()
          }
          frame "儲存檔案" {
            n151 = local read "file (use dialog)"() -> (w235:path)
            n152 = call <userlib>:"FGV_Data.vi"("Action_Data"=Control_Data."Idle") -> ("Data Array out"=w234:cluster{"Data name":string, "Data":variant}[])  [unwired: 7 in, 3 out]
            n153 = Write to Binary File(file (use dialog)=w235, data=w234) -> ()  [unwired: 4 in, 3 out]
          }
        }
      }
    }
    "error out" <- w68
  }
  n154 = local read "Project"() -> (w6:string)
  n155 = local read "Cluster In"() -> (w5:T1)
  n156 = Bundle("Project"=w6, "Cluster In"=w5) -> (w4:cluster{"Project":string, "Cluster In":T1})  [unwired: 1 in]
  n157 = To Variant(anything=w4) -> (Variant=w2:variant)
  n158 = Bundle("Project"=w6, "Variant"=w2) -> (w1:cluster{"Project":string, "Variant":variant})  [unwired: 1 in]
  n159 = call <userlib>:"FGV_Data.vi"("Action_Data"=Control_Data."Set Data", "Data In"=w1, "Data name"=w6) -> ()  [unwired: 5 in, 4 out]
